vi "Change Stream.vi"(11 "Index":dbl) -> ()   [LabVIEW 2019]
uses:
  <vilib>/Rock Robotics/Network Tables/NT Write Number.vi
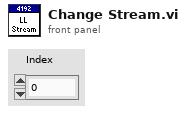
[diagram p1: front panel]
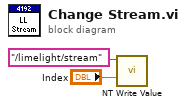
[diagram p0: block diagram]
diagram:
  n1 = call-poly <vilib>:"NT Write Value.vi"("Numeric"="Index", "Name"="/limelight/stream") -> ()  [unwired: 9 in, 1 out]
